vi "Untitled 1.vi"() -> ()   [LabVIEW 2014]
uses:
  Private/Class/meth.Constructor.vi
  Private/Class/meth.Destructor.vi
  GLue.lvlib
panel:
  out "Return Data":variant
  out "error out":errorcluster
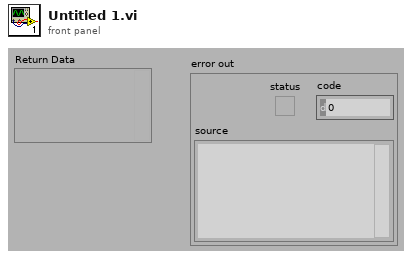
[diagram p1: front panel]
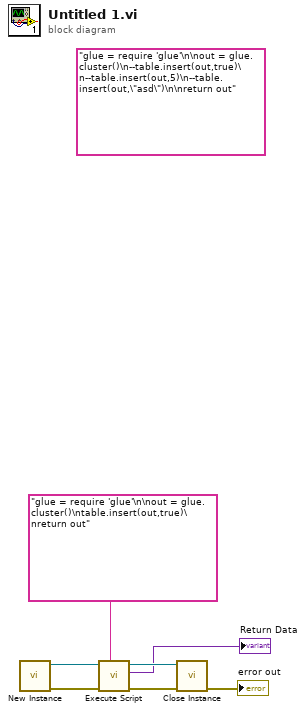
[diagram p0: block diagram]
diagram:
  (unwired) "glue = require 'glue'\n\nout = glue.cluster()\n--table.insert(out,true)\n--table.insert(out,5)\n--table.insert(out,\"asd\")\n\nreturn out" ("Script")
  n1 = call "New Instance.vi"() -> ("error out"=w3:errorcluster, "GLue out"=w4:refnum<class "class.GLue.lvclass">)  [unwired: 10 in]
  n2 = call "Execute Script.vi"("Script"="glue = require 'glue'\n\nout = glue.cluster()\ntable.insert(out,true)\nreturn out", "error in"=w3, "GLue in"=w4) -> ("error out"=w5:errorcluster, "Return Data"=→"Return Data":variant, "GLue out"=w6:refnum<class "class.GLue.lvclass">)  [unwired: 6 in]
  n3 = call "Close Instance.vi"("error in"=w5, "GLue in"=w6) -> ("error out"=→"error out":errorcluster)  [unwired: 9 in]
